vi "Insert visits.vi"(8 "Error In":errorcluster, 11 "Visits":T1 {"TotalSpend" format="£%.2g"; "SpendTaxedA" format="£%.2g"; "SpendTaxedB" format="£%.2g"}) -> (0 "Error Out":errorcluster, 2 "idvisits":i32, 3 "Output Data":string[][](array[string]))   [LabVIEW 2018, in "Database.lvlib"]
uses:
  Database.lvlib
  Visits--cluster.ctl
panel:
  out "Query [Debug]":string
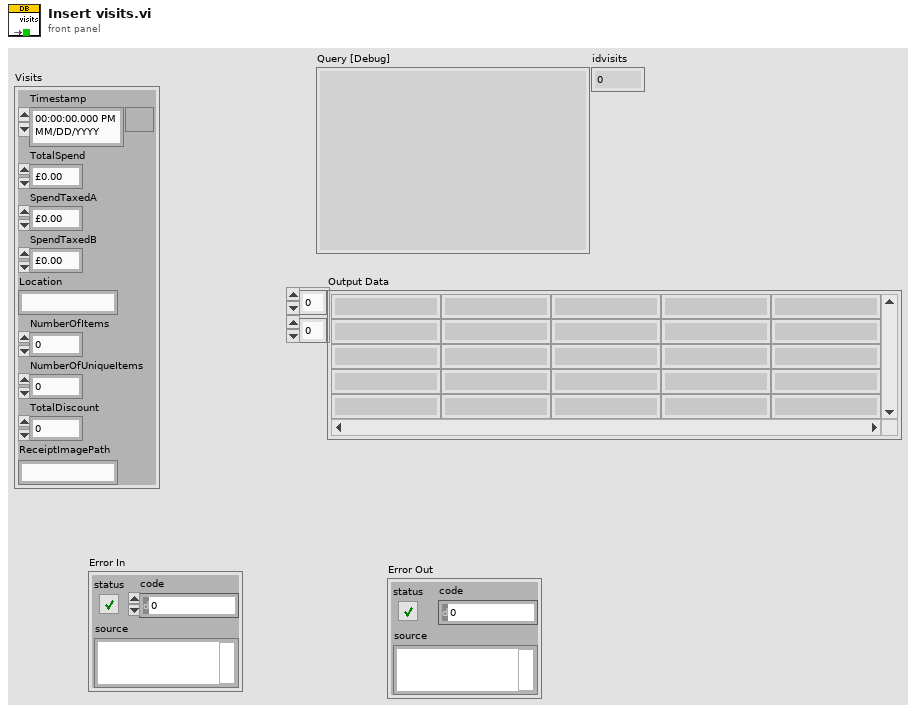
[diagram p1: front panel]
types:
  T1 = typedef "Database.lvlib/Visits--cluster.ctl" = cluster{"Timestamp":timestamp, "TotalSpend":dbl, "SpendTaxedA":dbl, "SpendTaxedB":dbl, "Location":string, "NumberOfItems":i32, "NumberOfUniqueItems":i32, "TotalDiscount":dbl, "ReceiptImagePath":string}
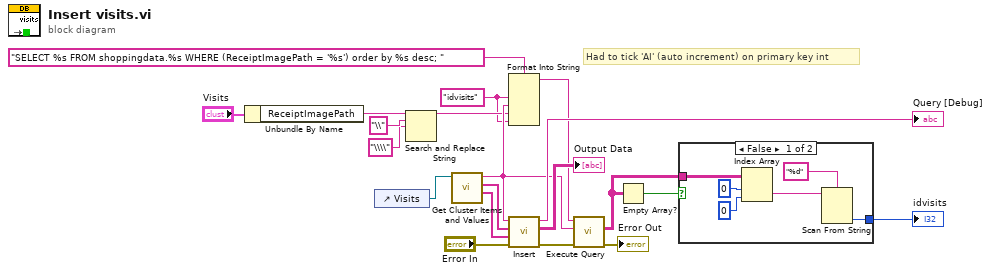
[diagram p0: block diagram]
diagram:
  w5 = "idvisits" ("input 1")
  # "Had to tick 'AI' (auto increment) on primary key int"
  n1 = Unbundle By Name("Visits") -> ("ReceiptImagePath"=w11:string)
  n2 = control-ref of="Visits"() -> (w20:refnum<vi>)
  n3 = Search and Replace String(input string=w11, search string="\\", replace string="\\\\" ("replace string (\"\")")) -> (result string=w6:string)  [unwired: 5 in, 3 out]
  n4 = call "Get Cluster Items and Values.vi"("Generic Cluster Reference"=w20) -> ("String Values"=w15:string[], "Column"=w16:string[], "Table"=w7:string)  [unwired: 7 in, 1 out]
  n5 = Format Into String(format string="SELECT %s FROM shoppingdata.%s WHERE (ReceiptImagePath = '%s') order by %s desc; ", w5, w7, w6, w5) -> (resulting string=w4:string)  [unwired: 2 in, 1 out]
  n6 = call "Insert.vi"("error in (no error)"="Error In", "String Values"=w15, "Columns"=w16, "Table"=w7) -> ("error out"=w14:errorcluster, "Output Data"=→"Output Data":string[][], "Query [Debug]"=→"Query [Debug]":string)  [unwired: 5 in]
  n7 = call "Execute Query.vi"("Error In"=w14, "Table"=w7, "Query"=w4) -> ("Error Out"=→"Error Out":errorcluster, "Output Data"=w3:string[][])  [unwired: 6 in, 1 out]
  n8 = Empty Array?(array=w3) -> (empty?=w2:bool)
  n9 = case shown="False" w2 {
    tunnel: w3 -> [w24 _]
    tunnel: [w21 _] -> w1
    frame False {
      n10 = Index Array(array=w24, index (row)=0 ("disabled index (row)"), index (col)=0 ("disabled index (col)")) -> (element=w22:string)
      n11 = Scan From String(format string="%d", input string=w22) -> (output 1=w21:i32)  [unwired: 3 in, 3 out]
    }
    frame True {
    }
  }
  "idvisits" <- w1
